vi "LED Globals.vi"() -> ()   [LabVIEW 2017]
uses:
  LED Notifier.ctl
  LED Control Type.ctl
panel:
  in  "LED Execute Notifier":refnum<notifier>
  in  "LED Set Notifier":refnum<notifier>
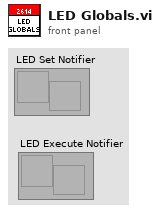
[diagram p1: front panel]
diagram:
